vi "libc path.vi"(8 "error in (no error)":errorcluster) -> (0 "error out":errorcluster, 3 "Path":path)   [LabVIEW 2013, in "Linux RT Utilities.lvlib"]
doc: "Path to glibc."
uses:
  Linux RT Utilities.lvlib
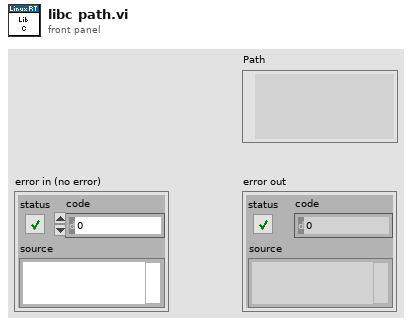
[diagram p1: front panel]
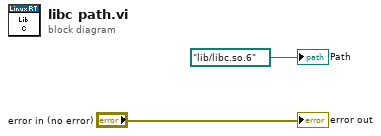
[diagram p0: block diagram]
diagram:
  "error out" <- "error in (no error)"
  "Path" <- path "/lib/libc.so.6" ("Path")
